vi "Enter_UnRock_Data.vi"() -> ()   [LabVIEW 2019]
uses:
  Calibration.ctl
  <vilib>/Utility/NIReport.llb/Report Type.ctl
  <vilib>/addons/database/Connection.llb/DB Tools Open Connec (Path).vi
  <vilib>/addons/_office/word.llb/Word Find & Replace (str).vi
  <vilib>/addons/database/_DB Variant To Data/Database Variant To Data.xnode
  <vilib>/Utility/NIReport.llb/NI_report.lvclass
  <vilib>/addons/database/NI_Database_API.lvlib
  TEST.lvclass
  <vilib>/Utility/NIReport.llb/NI_ReportGenerationCore.lvlib
  <vilib>/addons/_office/NI_ReportGenerationToolkit.lvlib
  <vilib>/Utility/NIReport.llb/Word/NI_Word.lvclass
panel:
  in  "校准日期":timestamp format="%<%Y/%m/%d>T"
  in  "生产日期":timestamp format="%<%Y/%m/%d>T"
  in  "批号":string
  in  "data":sgl[][](array[numeric]) format="%#.4g"
  out "初始化成功":bool
  out "error out":errorcluster
  in  "init":bool
  in  "NAME":string
  out "HS2":string[](array[string])
  out "CFXWC":string[](array[string])
  out "HAWC":string[](array[string])
  out "允许误差%":string[](array[string])
  out "试验力N(kg/g)":string[](array[string])
  out "执行状态":bool
  out "数据写入成功":bool
  in  "print_calibration":bool
  in  "print_data":bool
  in  "核验员":string
  in  "tsd":sgl[](array[numeric])=[1.0, 1.0, 1.0, 1.0] format="%#.4g"
  in  "停止":bool
  in  "write":bool
  in  "clear":bool
  in  "TEMP":string
  in  "TSN":string
  in  "MODE":string
  out "REP":sgl[](array[numeric]) format="%#.2g"
  out "HV":sgl[](array[numeric]) format="%#.2g"
  out "AVG":sgl[](array[numeric]) format="%#.2g"
  in  "TV":sgl[][](array[numeric]) format="%#.2g"
  in  "HS":sgl[](array[numeric])=[0.0, 0.0, 0.0, 0.0, 0.0] format="%#.2g"
  in  "HN":string[](array[string])
  in  "DIN":string
  out "Inacc":sgl[](array[numeric]) format="%#.2g"
  out "Dev":sgl[](array[numeric]) format="%#.4g"
  # "产品名称(首填)："
  # "型号："
  # "制造编号："
  # "温度："
  # "℃"
  # "试验力测试"
  # "最大偏差"
  # "误差%"
  # "2"
  # "3"
  # "1"
  # "测试力标准值"
  # "±"
  # "±"
  # "±"
  # "±"
  # "±"
  # "±"
  # "±"
  # "±"
  # "硬度测试"
  # "金刚石压头编号："
  # "测试值"
  # "硬度块\n标准值"
  # "硬度块\n  编号"
  # "硬度值"
  # "重复性"
  # "平均值"
  # "1"
  # "2"
  # "4"
  # "5"
  # "3"
  # "实际误差"
  # "允许误差"
  # "实际误差"
  # "允许误差"
  # "±1.0"
  # "1.0RA"
  # "RA"
  # "±1.5"
  # "1.5RB"
  # "RB"
  # "±1.5"
  # "1.5RC"
  # "RC"
  # "±1.2"
  # "1.2RC"
  # "RC"
  # "±1.0"
  # "1.2RC"
  # "RC"
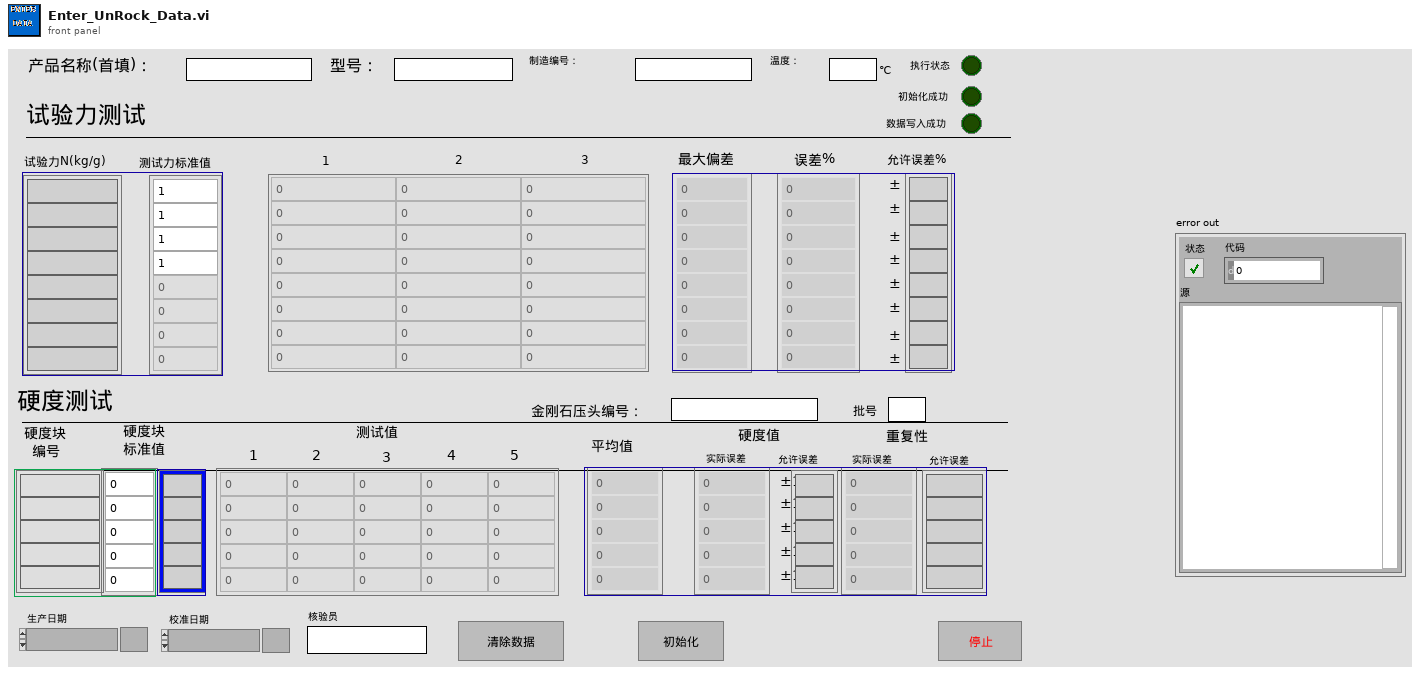
[diagram p1: front panel]
types:
  T1 = enum8{"Enabled", "Disabled", "Disabled and Grayed Out"}
  T2 = enum16{"open", "replace", "create", "open or create", "replace or create", "replace or create with confirmation"}
  T3 = typedef "TEST.lvclass/Calibration.ctl" = cluster{"NAM":string, "MODE":string, "TSN":string, "TDN":string, "DIN":string, "PROD":string, "CALD":string, "REV":string}
  T4 = typedef "NI_ReportGenerationCore.lvlib/Report Type.ctl" = enum16{"HTML", "Word", "Excel"}
  T5 = enum16{"maximized", "minimized", "normal", "no change"}
  T6 = typedef "NI_Database_API.lvlib/Conn ObjectReference.ctl" = refnum<k1>
  T7 = typedef "NI_Database_API.lvlib/DB Tools DataTypes.ctl" = enum16{"String", "Long (I32)", "Single (SGL)", "Double (DBL)", "Date/Time", "Binary"}
  T8 = cluster{"name":string, "database data type":T7, "defined size":i32}[]
  T9 = cluster{"name":string, "database data type":T7, "defined size":i32, bool}
  T10 = typedef "TEST.lvclass/Unrock_Cluster.ctl" = cluster{"MODE":string, "TSN":string, "Temp":string, "Test_load_row1":T11, "Test_load_row2":T11, "Test_load_row3":T11, "Test_load_row4":T11, "Test_load_row5":T11, "Test_load_row6":T11, "Test_load_row7":T11, "Test_load_row8":T11, "DIN":string, "Hardness_test_row1":T12, "Hardness_test_row2":T12, "Hardness_test_row3":T12, "Hardness_test_row4":T12, "Hardness_test_row5":T12}
  T11 = typedef "TEST.lvclass/Test_load.ctl" = cluster{"TEST1":sgl, "TEST2":sgl, "TEST3":sgl, "DEV":sgl, "INACC":sgl}
  T12 = typedef "TEST.lvclass/Hardness_test.ctl" = cluster{"HN":string, "HS":sgl, "TV1":sgl, "TV2":sgl, "TV3":sgl, "TV4":sgl, "TV5":sgl, "AVG":sgl, "HV":sgl, "REP":sgl}
  T13 = typedef "TEST.lvclass/Unrock_Data.ctl" = cluster{"MOD":string, "TSN":string, "Temp":string, "TEST1":sgl, "TEST2":sgl, "TEST3":sgl, "DEV":sgl, "INACC":sgl, "TEST1":sgl, "TEST2":sgl, "TEST3":sgl, "DEV":sgl, "INACC":sgl, "TEST1":sgl, "TEST2":sgl, "TEST3":sgl, "DEV":sgl, "INACC":sgl, "TEST1":sgl, "TEST2":sgl, "TEST3":sgl, "DEV":sgl, "INACC":sgl, "TEST1 5":sgl, "TEST2 5":sgl, "TEST3 5":sgl, "DEV 5":sgl, "INACC 5":sgl, "TEST1 4":sgl, "TEST2 4":sgl, "TEST3 4":sgl, "DEV 4":sgl, "INACC 4":sgl, "TEST1 3":sgl, "TEST2 3":sgl, "TEST3 3":sgl, "DEV 3":sgl, "INACC 3":sgl, "TEST1 2":sgl, "TEST2 2":sgl, "TEST3 2":sgl, "DEV 2":sgl, "INACC 2":sgl, "DIN":string, "HN":string, "HS":sgl, "TV1":sgl, "TV2":sgl, "TV3":sgl, "TV4":sgl, "TV5":sgl, "AVG":sgl, "HV":sgl, "REP":sgl, "HN":string, "HS":sgl, "TV1":sgl, "TV2":sgl, "TV3":sgl, "TV4":sgl, "TV5":sgl, "AVG":sgl, "HV":sgl, "REP":sgl, "HN":string, "HS":sgl, "TV1":sgl, "TV2":sgl, "TV3":sgl, "TV4":sgl, "TV5":sgl, "AVG":sgl, "HV":sgl, "REP":sgl, "HN":string, "HS":sgl, "TV1":sgl, "TV2":sgl, "TV3":sgl, "TV4":sgl, "TV5":sgl, "AVG":sgl, "HV":sgl, "REP":sgl, "HN":string, "HS":sgl, "TV1":sgl, "TV2":sgl, "TV3":sgl, "TV4":sgl, "TV5":sgl, "AVG":sgl, "HV":sgl, "REP":sgl, "NAM":string, "TDN":string, "PROD":string, "CALD":string, "REV":string}
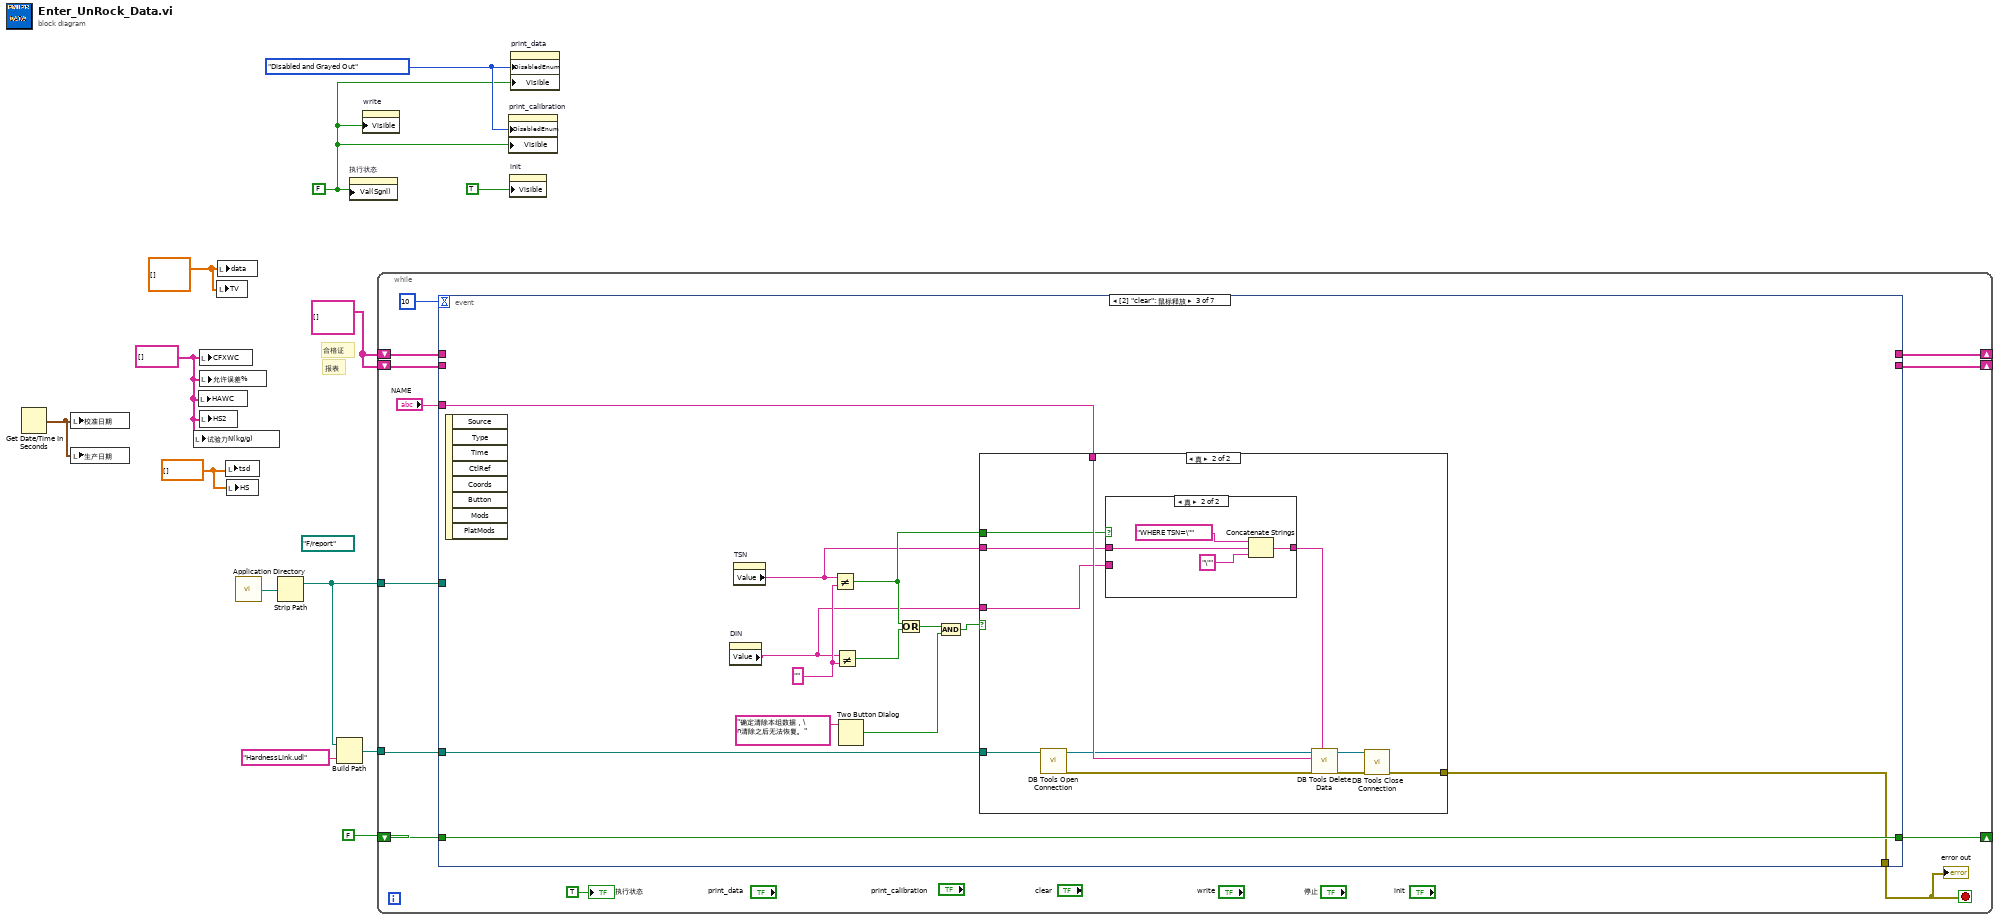
[diagram p0: block diagram]
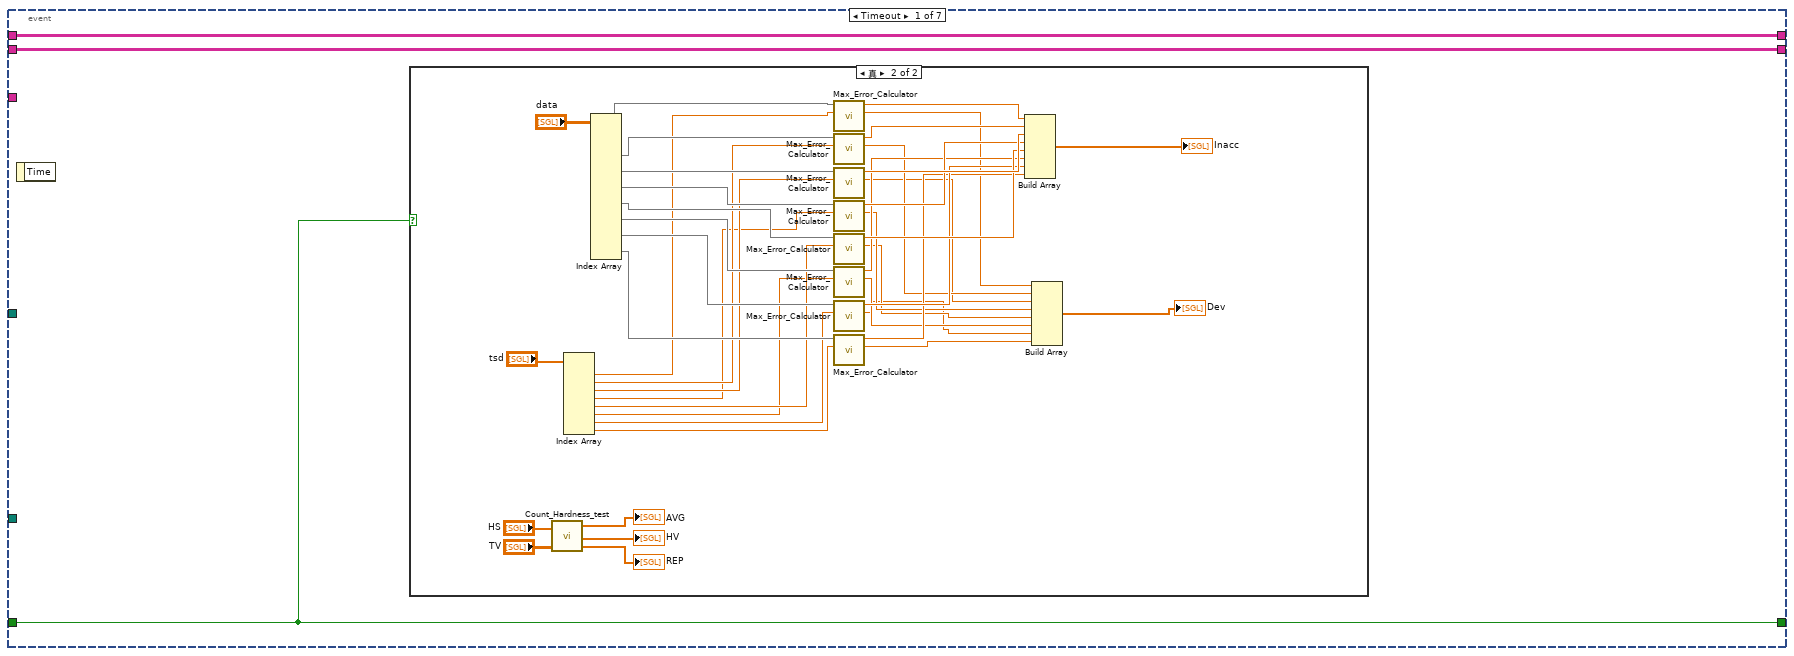
[diagram p2: hidden frame]
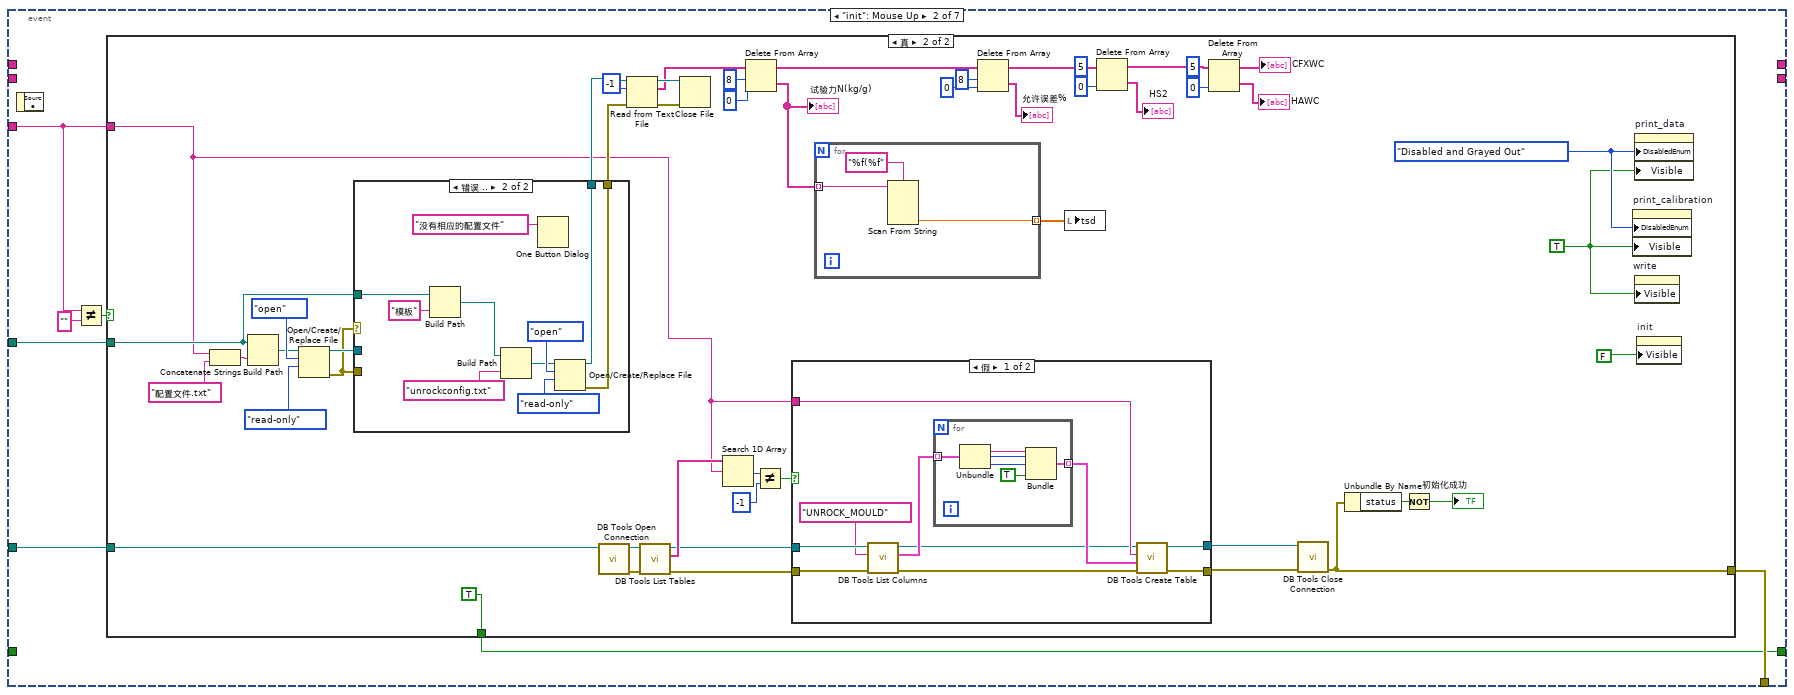
[diagram p4: hidden frame]
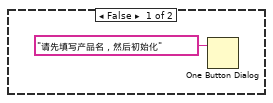
[diagram p5: hidden frame]
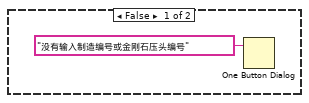
[diagram p8: hidden frame]
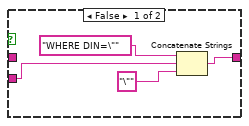
[diagram p9: hidden frame]
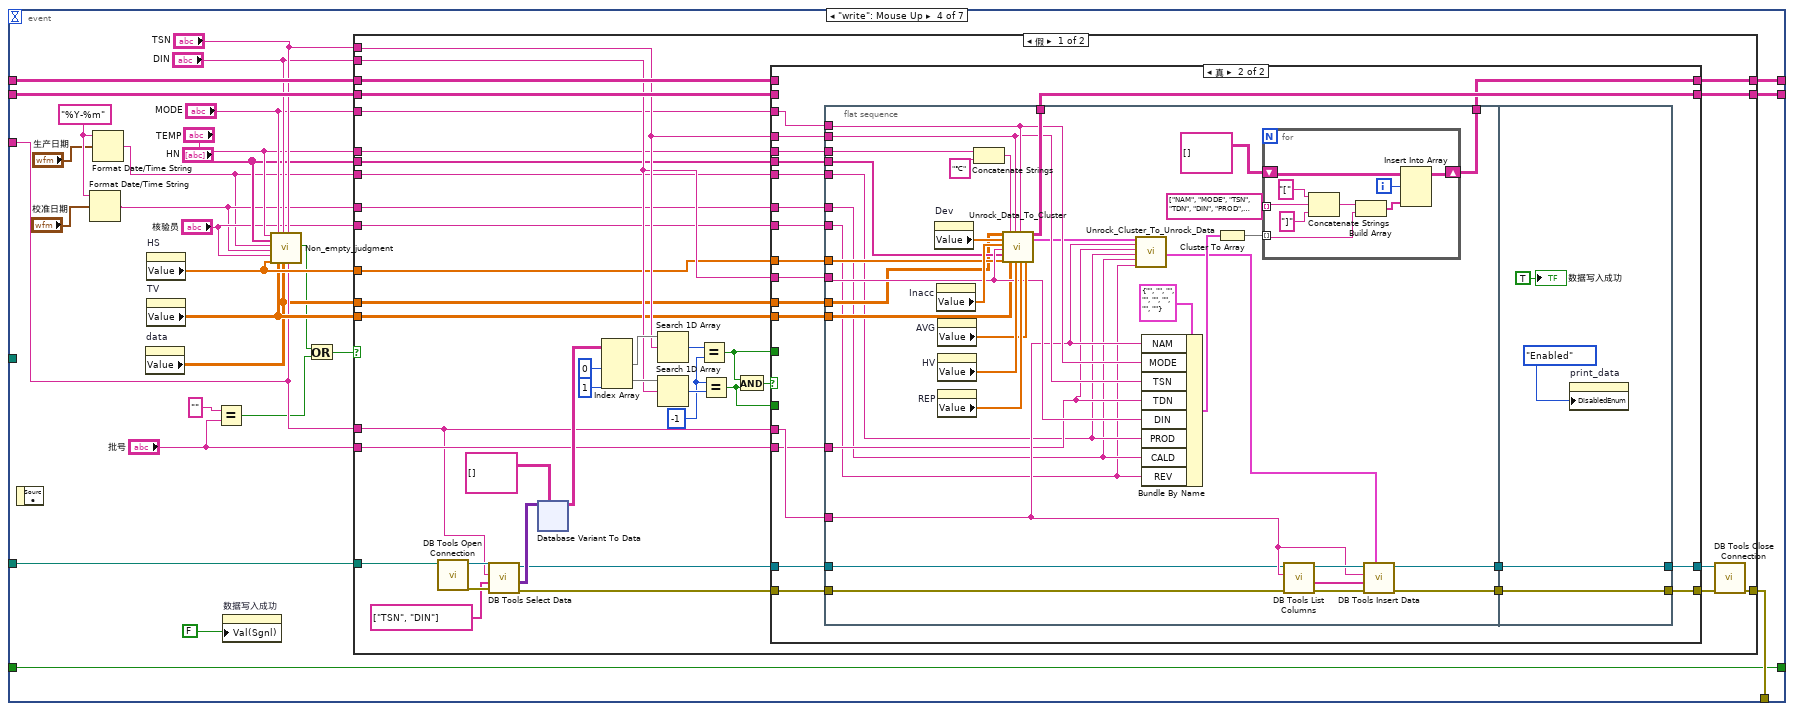
[diagram p10: hidden frame]
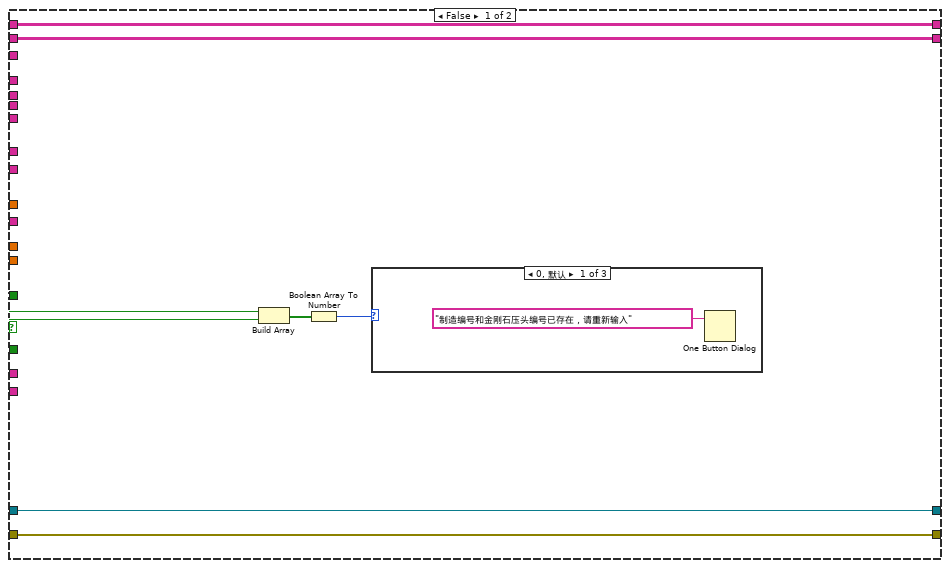
[diagram p11: hidden frame]
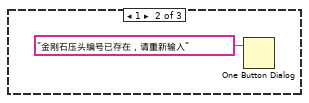
[diagram p12: hidden frame]
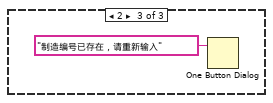
[diagram p13: hidden frame]
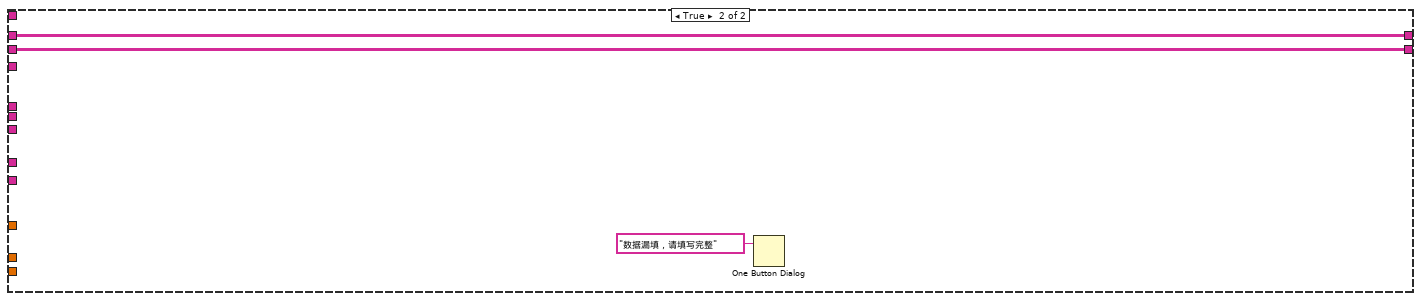
[diagram p14: hidden frame]
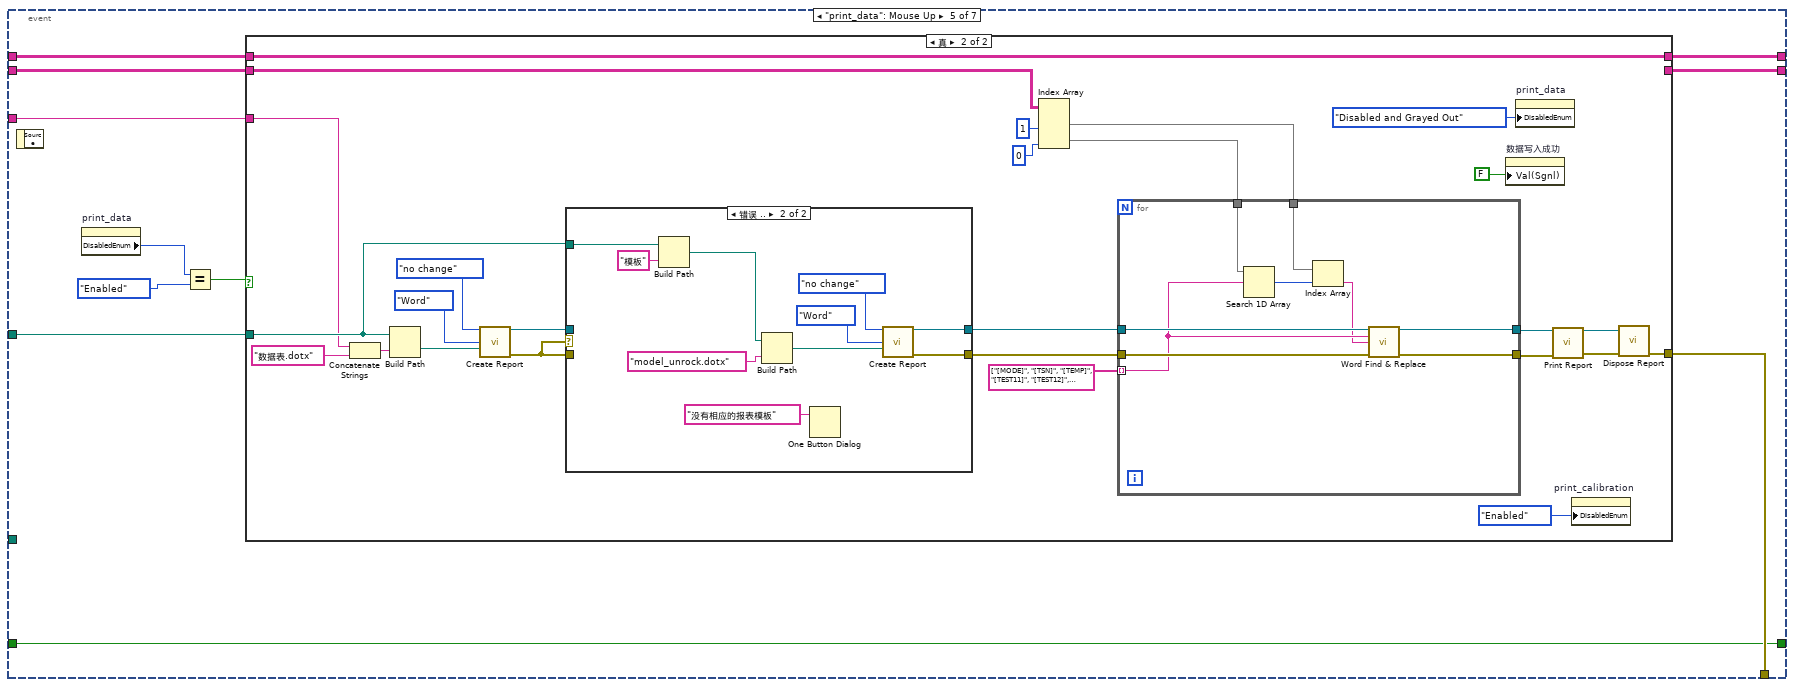
[diagram p15: hidden frame]
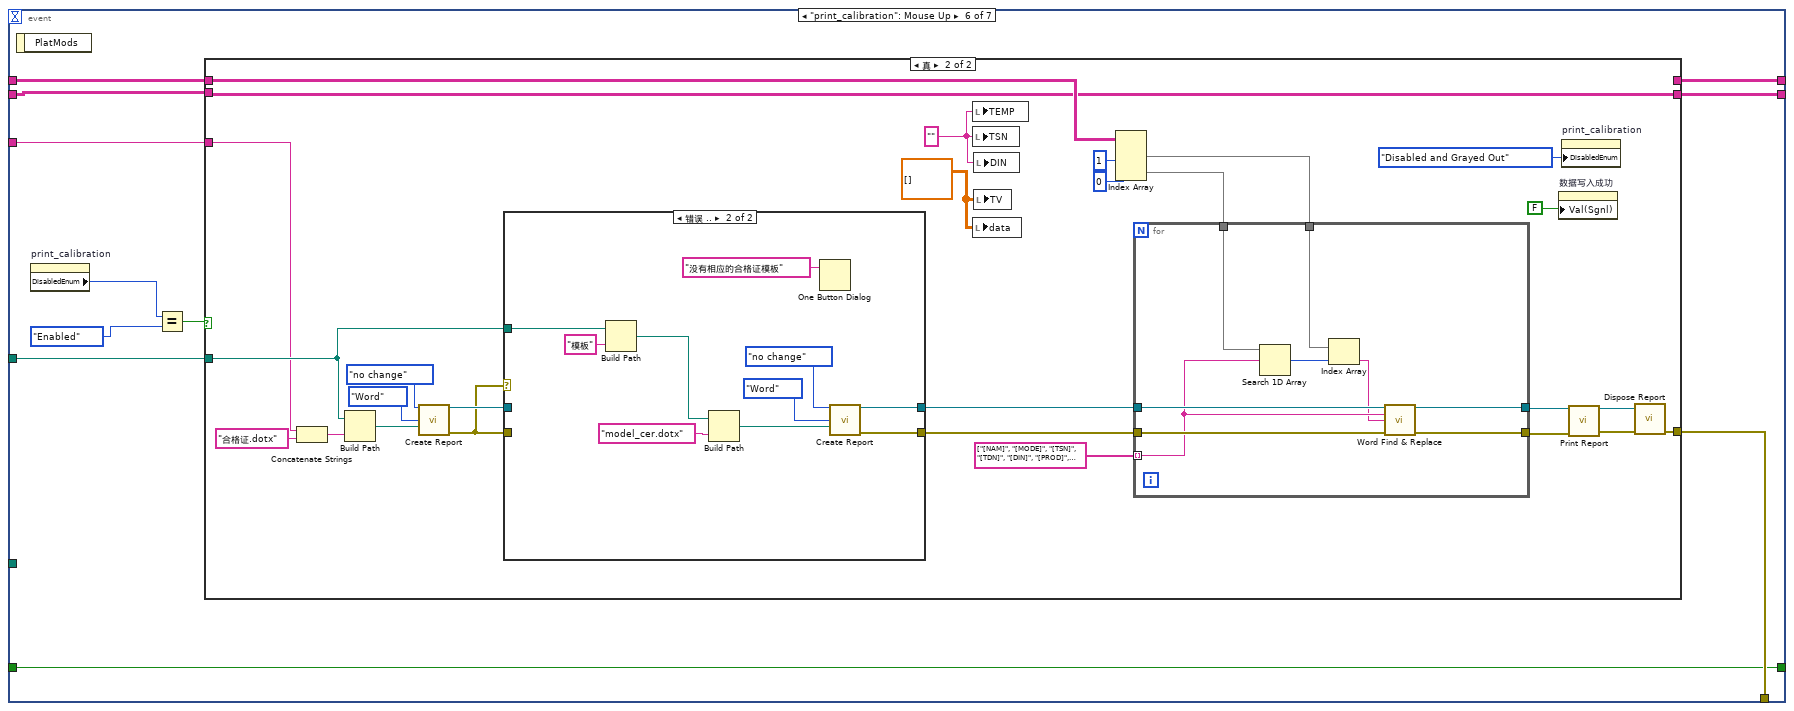
[diagram p18: hidden frame]
diagram:
  w6 = dbl[][] []
  w7 = sgl[] []
  w9 = string[] []
  (unwired) path "F:/report" ("data__in")
  w10 = FALSE
  w13 = T1."Disabled and Grayed Out" ("禁用")
  w12 = string[][] []
  # "报表"
  # "合格证"
  n1 = Get Date/Time In Seconds() -> (seconds since 1Jan1904=w1:timestamp)
  n2 = local write "校准日期"(w1) -> ()
  n3 = local write "生产日期"(w1) -> ()
  n4 = local write "试验力N(kg/g)"(w9) -> ()
  n5 = local write "HAWC"(w9) -> ()
  n6 = local write "CFXWC"(w9) -> ()
  n7 = local write "允许误差%"(w9) -> ()
  n8 = local write "HS2"(w9) -> ()
  n9 = local write "TV"(w6) -> ()
  n10 = local write "data"(w6) -> ()
  n11 = local write "tsd"(w7) -> ()
  n12 = local write "HS"(w7) -> ()
  n13 = call <vilib>:"Application Directory.vi"() -> ("Application Directory"=w5:path)
  n14 = Strip Path(path=w5) -> (stripped path=w2:path)  [unwired: 1 out]
  n15 = Build Path(base path=w2, name or relative path="HardnessLink.udl" ("名称或相对路径")) -> (appended path=w3:path)
  n16 = property on="执行状态" class="Bool (严格)"("Val(Sgnl)"=w10) -> ()  [unwired: 2 in, 2 out]
  n17 = property on="write" class="Bool (严格)"("Visible"=w10) -> ()  [unwired: 2 in, 2 out]
  n18 = while {
    shift-right: [w24] -> _
    shift-left: w12 -> [w23]
    shift-right: [w21] -> _
    shift-left: w12 -> [w20]
    tunnel: w2 -> [w15]
    shift-right: [w17] -> _
    shift-left: FALSE -> [w16]
    tunnel: w3 -> [w14]
    stop <- w18 stop-if-true
    n19 = event shown="[2] \"clear\": 鼠标释放" {
      selector: _ -> [_ _ _ _ _ _ _]
      dyn-events: _ -> [_ _ _ _ _ _ _]
      timeout: 10 -> [_ _ _ _ _ _ _]
      tunnel: [_ w75 w167 w217 w399 w459 errorcluster {"status"=TRUE, "code"=0, "source"=""} ("error out")] -> w18
      tunnel: [w28 _ _ w221 w391 w453 _] -> w24
      tunnel: w23 -> [w28 _ _ w218 w395 w454 _]
      tunnel: [w27 _ _ w220 w389 w452 _] -> w21
      tunnel: w20 -> [w27 _ _ w219 w390 w455 _]
      tunnel: "NAME" -> [_ w74 w169 w208 w397 w456 _]
      tunnel: w15 -> [_ w76 _ _ w398 w458 _]
      tunnel: [w26 w71 w173 w207 w396 w457 FALSE] -> w17
      tunnel: w16 -> [w26 _ w173 w207 w396 w457 _]
      tunnel: w14 -> [_ w70 w168 w199 _ _ _]
      event Timeout {
        n20 = event-data() -> ()  [unwired: 1 in, 1 out]
        n21 = case shown="真" w26 {
          frame False {
          }
          frame True {
            n22 = call "Count_Hardness_test.vi"("HS"="HS", "TV"="TV") -> ("AVG"=→"AVG":sgl[], "HV"=→"HV":sgl[], "REP"=→"REP":sgl[])
            n23 = Index Array(array="tsd") -> (element #1=w54:sgl, element #2=w53:sgl, element #3=w52:sgl, element #4=w51:sgl, element #5=w50:sgl, element #6=w49:sgl, element #7=w48:sgl, element #8=w47:sgl)  [unwired: 8 in]
            n24 = Index Array(array="data") -> (element #1=w63:sgl[], element #2=w62:sgl[], element #3=w61:sgl[], element #4=w60:sgl[], element #5=w59:sgl[], element #6=w58:sgl[], element #7=w57:sgl[], element #8=w56:sgl[])  [unwired: 16 in]
            n25 = call "Max_Error_Calculator.vi"("数值"=w54, "数组"=w63) -> ("dev"=w37:sgl, "inaccc"=w46:sgl)  [unwired: 8 in]
            n26 = call "Max_Error_Calculator.vi"("数值"=w53, "数组"=w62) -> ("dev"=w36:sgl, "inaccc"=w45:sgl)  [unwired: 8 in]
            n27 = call "Max_Error_Calculator.vi"("数值"=w52, "数组"=w61) -> ("dev"=w35:sgl, "inaccc"=w44:sgl)  [unwired: 8 in]
            n28 = call "Max_Error_Calculator.vi"("数值"=w51, "数组"=w60) -> ("dev"=w34:sgl, "inaccc"=w43:sgl)  [unwired: 8 in]
            n29 = call "Max_Error_Calculator.vi"("数值"=w50, "数组"=w59) -> ("dev"=w33:sgl, "inaccc"=w42:sgl)  [unwired: 8 in]
            n30 = call "Max_Error_Calculator.vi"("数值"=w49, "数组"=w58) -> ("dev"=w32:sgl, "inaccc"=w41:sgl)  [unwired: 8 in]
            n31 = call "Max_Error_Calculator.vi"("数值"=w48, "数组"=w57) -> ("dev"=w31:sgl, "inaccc"=w40:sgl)  [unwired: 8 in]
            n32 = call "Max_Error_Calculator.vi"("数值"=w47, "数组"=w56) -> ("dev"=w30:sgl, "inaccc"=w39:sgl)  [unwired: 8 in]
            n33 = Build Array(w46, w45, w44, w43, w42, w41, w40, w39) -> (→"Inacc":sgl[])
            n34 = Build Array(w37, w36, w35, w34, w33, w32, w31, w30) -> (→"Dev":sgl[])
          }
        }
      }
      event "init": Mouse Up {
        n35 = event-data() -> ()  [unwired: 1 in, 1 out]
        n36 = Not Equal?(x=w74, y="" ("NAME")) -> (x != y?=w72:bool)
        n37 = case shown="真" w72 {
          tunnel: w70 -> [_ w127]
          tunnel: w76 -> [_ w90]
          tunnel: [_ w89] -> w75
          tunnel: w74 -> [_ w78]
          tunnel: [_ TRUE] -> w71
          frame False {
            n38 = One Button Dialog(message="请先填写产品名，然后初始化" ("消息")) -> ()  [unwired: 1 in, 1 out]
          }
          frame True {
            w115 = T1."Disabled and Grayed Out" ("禁用")
            w114 = TRUE ("可见")
            n39 = Concatenate Strings(w78, "配置文件.txt" ("名称或相对路径")) -> (w95:string)
            n40 = Build Path(base path=w90, name or relative path=w95) -> (appended path=w108:path)
            n41 = Open/Create/Replace File(file path (use dialog)=w108, operation (0:open)=T2."open" ("操作(0:open)"), access (0:read/write)=enum16{"read/write", "read-only", "write-only"}."read-only" ("权限(0:read/write)")) -> (refnum out=w93:refnum<file>, error out=w91:errorcluster)  [unwired: 3 in, 1 out]
            n42 = case shown="错误 .." w91 {
              tunnel: [w132 w142] -> w94
              tunnel: w93 -> [w132 _]
              tunnel: [w131 w141] -> w92
              tunnel: w91 -> [w131 _]
              tunnel: w90 -> [_ w136]
              frame No Error {
              }
              frame Error {
                n43 = Build Path(base path=w136, name or relative path="模板" ("名称或相对路径")) -> (appended path=w134:path)
                n44 = Build Path(base path=w134, name or relative path="unrockconfig.txt") -> (appended path=w138:path)
                n45 = One Button Dialog(message="没有相应的配置文件" ("消息")) -> ()  [unwired: 1 in, 1 out]
                n46 = Open/Create/Replace File(file path (use dialog)=w138, operation (0:open)=T2."open" ("操作(0:open)"), access (0:read/write)=enum16{"read/write", "read-only", "write-only"}."read-only" ("权限(0:read/write)")) -> (refnum out=w142:refnum<file>, error out=w141:errorcluster)  [unwired: 3 in, 1 out]
              }
            }
            n47 = call-poly <vilib>:"DB Tools Open Connection.vi"("connection information"=w127) -> ("error out"=w125:errorcluster, "connection reference"=w126:T6)  [unwired: 7 in]
            n48 = Read from Text File(file (use dialog)=w94, count=-1 ("计数"), error in=w92) -> (refnum out=w110:refnum<file>, text=w107:string[], error out=w111:errorcluster)  [unwired: 1 in, 1 out]
            n49 = call <vilib>:"DB Tools List Tables.vi"("error in (no error)"=w125, "connection reference"=w126) -> ("error out"=w119:errorcluster, "tables"=w124:string[], "connection reference out"=w120:T6)  [unwired: 3 in]
            n50 = Close File(refnum=w110, error in=w111) -> ()  [unwired: 2 out]
            n51 = Search 1D Array(1D array=w124, element=w78) -> (index of element=w123:i32)  [unwired: 1 in]
            n52 = Delete From Array(array=w107, length=8 ("长度"), index=0 ("索引")) -> (deleted portion=w85:string[], array with subset deleted=w79:string[])
            "试验力N(kg/g)" <- w85
            n53 = Not Equal?(x=w123, y=-1) -> (x != y?=w121:bool)
            n54 = case shown="假" w121 {
              tunnel: [w144 w160] -> w117
              tunnel: w120 -> [w152 w160]
              tunnel: w119 -> [w151 w159]
              tunnel: [w143 w159] -> w118
              tunnel: w78 -> [w147 _]
              frame False {
                n55 = call <vilib>:"DB Tools List Columns.vi"("error in (no error)"=w151, "table"="UNROCK_MOULD", "connection reference"=w152) -> ("error out"=w145:errorcluster, "column information"=w149:T8, "connection reference out"=w146:T6)  [unwired: 1 in, 1 out]
                n56 = for {
                  tunnel: w149 -> [w158] mode=indexing
                  tunnel: [w153] -> w148 mode=indexing
                  n57 = Unbundle(w158) -> ("name"=w157:string, "database data type"=w156:T7, "defined size"=w155:i32)
                  n58 = Bundle("name"=w157, "database data type"=w156, "defined size"=w155, TRUE) -> (w153:T9)  [unwired: 1 in]
                }
                n59 = call <vilib>:"DB Tools Create Table.vi"("error in (no error)"=w145, "column information"=w148, "table"=w147, "connection reference"=w146) -> ("error out"=w143:errorcluster, "connection reference out"=w144:T6)  [unwired: 4 in]
              }
              frame True {
              }
            }
            n60 = for {
              tunnel: w85 -> [w129] mode=indexing
              tunnel: [w128] -> w86 mode=indexing
              n61 = Scan From String(format string="%f(%f" ("格式字符串"), input string=w129) -> (output 2=w128:dbl)  [unwired: 5 in, 3 out]
            }
            n62 = Delete From Array(array=w79, length=8 ("长度"), index=0 ("索引")) -> (deleted portion=→"允许误差%":string[], array with subset deleted=w102:string[])
            n63 = local write "tsd"(w86) -> ()
            n64 = Delete From Array(array=w102, length=5 ("长度"), index=0 ("索引")) -> (deleted portion=→"HS2":string[], array with subset deleted=w99:string[])
            n65 = Delete From Array(array=w99, length=5 ("长度"), index=0 ("索引")) -> (deleted portion=→"HAWC":string[], array with subset deleted=→"CFXWC":string[])
            n66 = call <vilib>:"DB Tools Close Connection.vi"("error in (no error)"=w118, "connection reference"=w117) -> ("error out"=w89:errorcluster)  [unwired: 5 in]
            n67 = Unbundle By Name(w89) -> ("status"=w88:bool)
            n68 = Not(x=w88) -> (.not. x?=→"初始化成功":bool)
            n69 = property on="print_calibration" class="Bool (严格)"("DisabledEnum"=w115, "Visible"=w114) -> ()  [unwired: 2 in, 2 out]
            n70 = property on="print_data" class="Bool (严格)"("DisabledEnum"=w115, "Visible"=w114) -> ()  [unwired: 2 in, 2 out]
            n71 = property on="write" class="Bool (严格)"("Visible"=w114) -> ()  [unwired: 2 in, 2 out]
            n72 = property on="init" class="Bool (严格)"("Visible"=FALSE ("可见")) -> ()  [unwired: 2 in, 2 out]
          }
        }
      }
      event "clear": Mouse Up {
        w172 = ""
        n73 = event-data() -> ()  [unwired: 1 in, 8 out]
        n74 = property on="DIN" class="Str"() -> ("Value"=w165:string)  [unwired: 2 in, 2 out]
        n75 = property on="TSN" class="Str"() -> ("Value"=w166:string)  [unwired: 2 in, 2 out]
        n76 = Not Equal?(x=w166, y=w172) -> (x != y?=w170:bool)
        n77 = Not Equal?(x=w165, y=w172) -> (x != y?=w171:bool)
        n78 = Two Button Dialog(message="确定清除本组数据，\n清除之后无法恢复。" ("消息")) -> (T button?=w161:bool)  [unwired: 2 in]
        n79 = Or(x=w170, y=w171) -> (x .or. y?=w163:bool)
        n80 = And(x=w163, y=w161) -> (x .and. y?=w162:bool)
        n81 = case shown="真" w162 {
          tunnel: w168 -> [_ w185]
          tunnel: w169 -> [_ w184]
          tunnel: [_ w183] -> w167
          tunnel: w166 -> [_ w177]
          tunnel: w170 -> [_ w176]
          tunnel: w165 -> [_ w175]
          frame False {
            n82 = One Button Dialog(message="没有输入制造编号或金刚石压头编号" ("消息")) -> ()  [unwired: 1 in, 1 out]
          }
          frame True {
            n83 = call-poly <vilib>:"DB Tools Open Connection.vi"("connection information"=w185) -> ("error out"=w181:errorcluster, "connection reference"=w182:T6)  [unwired: 7 in]
            n84 = case shown="真" w176 {
              tunnel: [w187 w191] -> w178
              tunnel: w177 -> [_ w190]
              tunnel: w175 -> [w186 _]
              frame False {
                n85 = Concatenate Strings("WHERE DIN=\"", w186, "\"" ("字符串")) -> (w187:string)
              }
              frame True {
                n86 = Concatenate Strings("WHERE TSN=\"", w190, "\"" ("字符串")) -> (w191:string)
              }
            }
            n87 = call <vilib>:"DB Tools Delete Data.vi"("condition"=w178, "error in (no error)"=w181, "table"=w184, "connection reference"=w182) -> ("error out"=w180:errorcluster, "connection reference out"=w179:T6)  [unwired: 6 in]
            n88 = call <vilib>:"DB Tools Close Connection.vi"("error in (no error)"=w180, "connection reference"=w179) -> ("error out"=w183:errorcluster)  [unwired: 5 in]
          }
        }
      }
      event "write": Mouse Up {
        w198 = "%Y-%m" ("时间格式字符串(%c)")
        n89 = event-data() -> ()  [unwired: 1 in, 1 out]
        n90 = Format Date/Time String(time format string (%c)=w198, seconds (now)="校准日期") -> (date/time string=w195:string)  [unwired: 1 in]
        n91 = Format Date/Time String(time format string (%c)=w198, seconds (now)="生产日期") -> (date/time string=w194:string)  [unwired: 1 in]
        n92 = property on="data" class="Arr (严格)"() -> ("Value"=w205:sgl[][])  [unwired: 2 in, 2 out]
        n93 = property on="HS" class="Arr (严格)"() -> ("Value"=w210:sgl[])  [unwired: 2 in, 2 out]
        n94 = property on="TV" class="Arr (严格)"() -> ("Value"=w209:sgl[][])  [unwired: 2 in, 2 out]
        n95 = Equal?(x="", y="批号") -> (x = y?=w200:bool)
        n96 = property on="数据写入成功" class="Bool (严格)"("Val(Sgnl)"=FALSE) -> ()  [unwired: 2 in, 2 out]
        n97 = call "Non_empty_judgment.vi"("TEMP"="TEMP", "HN"="HN", "生产日期"=w194, "校准日期"=w195, "核验员"="核验员", "HS"=w210, "MODE"="MODE", "TV"=w209, "DIN"="DIN", "TESTS"=w205, "TSN"="TSN", "NAME"=w208) -> ("结果"=w201:bool)  [unwired: 7 in]
        n98 = Or(x=w201, y=w200) -> (x .or. y?=w202:bool)
        n99 = case shown="假" w202 {
          tunnel: [w260 w387] -> w221
          tunnel: [w259 w388] -> w220
          tunnel: w219 -> [w244 w388]
          tunnel: w218 -> [w243 w387]
          tunnel: w199 -> [w242 _]
          tunnel: [w235 _] -> w217
          tunnel: "TSN" -> [w234 _]
          tunnel: "DIN" -> [w233 _]
          tunnel: "MODE" -> [w232 _]
          tunnel: "TEMP" -> [w231 _]
          tunnel: "HN" -> [w230 _]
          tunnel: w194 -> [w229 _]
          tunnel: w195 -> [w228 _]
          tunnel: "核验员" -> [w227 _]
          tunnel: w210 -> [w226 _]
          tunnel: w209 -> [w225 _]
          tunnel: w208 -> [w222 _]
          tunnel: w205 -> [w224 _]
          tunnel: "批号" -> [w223 _]
          frame False {
            w246 = -1
            n100 = call-poly <vilib>:"DB Tools Open Connection.vi"("connection information"=w242) -> ("error out"=w257:errorcluster, "connection reference"=w258:T6)  [unwired: 7 in]
            n101 = call <vilib>:"DB Tools Select Data.vi"("error in (no error)"=w257, "columns"=string[] ["TSN", "DIN"], "table"=w222, "connection reference"=w258) -> ("error out"=w238:errorcluster, "data"=w255:variant[][], "connection reference out"=w239:T6)  [unwired: 2 in]
            n102 = xnode "Database Variant To Data"("database variant"=w255, "type"=string[][] []) -> ("data"=w253:string[][])  [unwired: 1 in, 1 out]
            n103 = Index Array(array=w253, index (col) #1=0 ("禁用的索引 (列)"), index (col) #2=1 ("索引 (列)")) -> (element #1=w250:string[], element #2=w249:string[])  [unwired: 2 in]
            n104 = Search 1D Array(1D array=w250, element=w234) -> (index of element=w248:i32)  [unwired: 1 in]
            n105 = Search 1D Array(1D array=w249, element=w233) -> (index of element=w247:i32)  [unwired: 1 in]
            n106 = Equal?(x=w248, y=w246) -> (x = y?=w241:bool)
            n107 = Equal?(x=w246, y=w247) -> (x = y?=w240:bool)
            n108 = And(x=w241, y=w240) -> (x .and. y?=w245:bool)
            n109 = case shown="真" w245 {
              tunnel: [w267 w292] -> w260
              tunnel: [w268 w291] -> w259
              tunnel: w234 -> [_ w290]
              tunnel: w233 -> [_ w289]
              tunnel: w244 -> [w268 _]
              tunnel: w243 -> [w267 _]
              tunnel: w222 -> [_ w288]
              tunnel: w241 -> [w265 _]
              tunnel: w240 -> [w266 _]
              tunnel: w239 -> [w262 w287]
              tunnel: w238 -> [w261 w286]
              tunnel: [w262 w284] -> w237
              tunnel: [w261 w282] -> w236
              tunnel: w232 -> [_ w281]
              tunnel: w231 -> [_ w280]
              tunnel: w230 -> [_ w279]
              tunnel: w229 -> [_ w278]
              tunnel: w226 -> [_ w277]
              tunnel: w225 -> [_ w276]
              tunnel: w228 -> [_ w275]
              tunnel: w227 -> [_ w274]
              tunnel: w224 -> [_ w273]
              tunnel: w223 -> [_ w272]
              frame False {
                n110 = Build Array(w265, w266) -> (w264:bool[])
                n111 = Boolean Array To Number(Boolean array=w264) -> (number=w263:u32)
                n112 = case shown="0, 默认" w263 {
                  frame 0, Default {
                    n113 = One Button Dialog(message="制造编号和金刚石压头编号已存在，请重新输入" ("消息")) -> ()  [unwired: 1 in, 1 out]
                  }
                  frame 1 {
                    n114 = One Button Dialog(message="金刚石压头编号已存在，请重新输入" ("消息")) -> ()  [unwired: 1 in, 1 out]
                  }
                  frame 2 {
                    n115 = One Button Dialog(message="制造编号已存在，请重新输入" ("消息")) -> ()  [unwired: 1 in, 1 out]
                  }
                }
              }
              frame True {
                n116 = flat-sequence {
                  tunnel: [w317] -> w292
                  tunnel: [w314] -> w291
                  tunnel: w290 -> [w304]
                  tunnel: w289 -> [w312]
                  tunnel: w288 -> [w299]
                  tunnel: w287 -> [w294]
                  tunnel: w286 -> [w293]
                  tunnel: [w311] -> w285
                  tunnel: [w310] -> w283
                  tunnel: w281 -> [w305]
                  tunnel: w280 -> [w309]
                  tunnel: w279 -> [w308]
                  tunnel: w278 -> [w297]
                  tunnel: w277 -> [w307]
                  tunnel: w276 -> [w306]
                  tunnel: w275 -> [w296]
                  tunnel: w274 -> [w295]
                  tunnel: w273 -> [w303]
                  tunnel: w272 -> [w298]
                  tunnel: w285 -> [w340]
                  tunnel: [w340] -> w284
                  tunnel: w283 -> [w339]
                  tunnel: [w339] -> w282
                  frame #0 {
                    n117 = property on="Dev" class="Arr (严格)"() -> ("Value"=w325:sgl[])  [unwired: 2 in, 2 out]
                    n118 = property on="Inacc" class="Arr (严格)"() -> ("Value"=w324:sgl[])  [unwired: 2 in, 2 out]
                    n119 = property on="AVG" class="Arr (严格)"() -> ("Value"=w321:sgl[])  [unwired: 2 in, 2 out]
                    n120 = property on="HV" class="Arr (严格)"() -> ("Value"=w323:sgl[])  [unwired: 2 in, 2 out]
                    n121 = property on="REP" class="Arr (严格)"() -> ("Value"=w322:sgl[])  [unwired: 2 in, 2 out]
                    n122 = Concatenate Strings(w309, "℃") -> (w319:string)
                    n123 = call "Unrock_Data_To_Cluster.vi"("Test"=w303, "Dev"=w325, "Inacc"=w324, "DIN"=w312, "HN"=w308, "HS"=w307, "TEMP"=w319, "TV"=w306, "TSN"=w304, "HV"=w323, "MODE"=w305, "REP"=w322, "AVG"=w321) -> ("All_data_String"=w317:string[][], "输出簇"=w301:T10)  [unwired: 5 in]
                    n124 = call "Unrock_Cluster_To_Unrock_Data.vi"("Unrock_Cluster"=w301, "NAM"=w299, "TDN"=w298, "PROD"=w297, "CALD"=w296, "REV"=w295) -> ("Cluster67"=w302:T13)  [unwired: 13 in]
                    n125 = Bundle By Name(cluster=T3 {"NAM"="", "MODE"="", "TSN"="", "TDN"="", "DIN"="", "PROD"="", "CALD"="", "REV"=""} ("Cal"), "NAM"=w299, "MODE"=w305, "TSN"=w304, "TDN"=w298, "DIN"=w312, "PROD"=w297, "CALD"=w296, "REV"=w295) -> (w313:T3)
                    n126 = Cluster To Array(cluster=w313) -> (array=w316:string[])
                    n127 = for {
                      tunnel: w316 -> [w337] mode=indexing
                      tunnel: string[] ["NAM", "MODE", "TSN", "TDN", "DIN", "PROD", "CALD", "REV"] ("columns 3") -> [w331] mode=indexing
                      shift-right: [w335] -> w314
                      shift-left: string[][] [] -> [w336]
                      i -> [w334]
                      n128 = Concatenate Strings("[" ("字符串"), w331, "]" ("字符串")) -> (w330:string)
                      n129 = Build Array(w330, w337) -> (w329:string[])
                      n130 = Insert Into Array(array=w336, index (row)=w334, new element=w329) -> (w335:string[][])  [unwired: 1 in]
                    }
                    n131 = call <vilib>:"DB Tools List Columns.vi"("error in (no error)"=w293, "table"=w299, "connection reference"=w294) -> ("error out"=w328:errorcluster, "columns"=w327:string[], "connection reference out"=w326:T6)  [unwired: 1 in, 1 out]
                    n132 = call <vilib>:"DB Tools Insert Data.vi"("data"=w302, "error in (no error)"=w328, "columns"=w327, "table"=w299, "connection reference"=w326) -> ("error out"=w310:errorcluster, "connection reference out"=w311:T6)  [unwired: 5 in]
                  }
                  frame #1 {
                    n133 = property on="print_data" class="Bool (严格)"("DisabledEnum"=T1."Enabled" ("禁用")) -> ()  [unwired: 2 in, 2 out]
                    "数据写入成功" <- TRUE
                  }
                }
              }
            }
            n134 = call <vilib>:"DB Tools Close Connection.vi"("error in (no error)"=w236, "connection reference"=w237) -> ("error out"=w235:errorcluster)  [unwired: 5 in]
          }
          frame True {
            n135 = One Button Dialog(message="数据漏填，请填写完整" ("消息")) -> ()  [unwired: 1 in, 1 out]
          }
        }
      }
      event "print_data": Mouse Up {
        n136 = event-data() -> ()  [unwired: 1 in, 1 out]
        n137 = property on="print_data" class="Bool (严格)"() -> ("DisabledEnum"=w393:T1)  [unwired: 2 in, 2 out]
        n138 = Equal?(x=w393, y=T1."Enabled" ("禁用")) -> (x = y?=w394:bool)
        n139 = case shown="真" w394 {
          tunnel: [_ w417] -> w399
          tunnel: w398 -> [_ w412]
          tunnel: w397 -> [_ w411]
          tunnel: w395 -> [w401 w408]
          tunnel: [w401 _] -> w391
          tunnel: w390 -> [w400 w403]
          tunnel: [w400 w403] -> w389
          frame False {
          }
          frame True {
            n140 = Concatenate Strings(w411, "数据表.dotx" ("字符串")) -> (w418:string)
            n141 = Build Path(base path=w412, name or relative path=w418) -> (appended path=w420:path)
            n142 = call <vilib>:"Create Report.vi"("window state (normal)"=T5."no change", "report type"=Report_Type."Word", "template (empty)"=w420) -> ("report out"=w413:refnum<class "NI_report.lvclass">, "error out"=w416:errorcluster)  [unwired: 11 in]
            n143 = case shown="错误 .." w416 {
              tunnel: w416 -> [w429 _]
              tunnel: [w429 w437] -> w415
              tunnel: [w428 w436] -> w414
              tunnel: w413 -> [w428 _]
              tunnel: w412 -> [_ w433]
              frame No Error {
              }
              frame Error {
                n144 = Build Path(base path=w433, name or relative path="模板" ("名称或相对路径")) -> (appended path=w431:path)
                n145 = Build Path(base path=w431, name or relative path="model_unrock.dotx") -> (appended path=w434:path)
                n146 = One Button Dialog(message="没有相应的报表模板" ("消息")) -> ()  [unwired: 1 in, 1 out]
                n147 = call <vilib>:"Create Report.vi"("window state (normal)"=T5."no change", "report type"=Report_Type."Word", "template (empty)"=w434) -> ("report out"=w436:refnum<class "NI_report.lvclass">, "error out"=w437:errorcluster)  [unwired: 11 in]
              }
            }
            n148 = Index Array(array=w408, index (col) #1=1 ("禁用的索引 (列)"), index (col) #2=0 ("索引 (列)")) -> (element #1=w404:string[], element #2=w405:string[])  [unwired: 2 in]
            n149 = for {
              tunnel: string[] ["[MODE]", "[TSN]", "[TEMP]", "[TEST11]", "[TEST12]", "[TEST13]", "[DEV1]", "[INACC1]", "[TEST21]", "[TEST22]", "[TEST23]", "[DEV2]", "[INACC2]", "[TEST31]", "[TEST32]", "[TEST33]", "[DEV3]", "[INACC3]", "[TEST41]", "[TEST42]", "[TEST43]", "[DEV4]", "[INACC4]", "[TEST51]", "[TEST52]", "[TEST53]", "[DEV5]", "[INACC5]", "[TEST61]", "[TEST62]", "[TEST63]", "[DEV6]", "[INACC6]", "[TEST71]", "[TEST72]", "[TEST73]", "[DEV7]", "[INACC7]", "[TEST81]", "[TEST82]", "[TEST83]", "[DEV8]", "[INACC8]", "[DIN]", "[HN1]", "[HS1]", "[TV11]", "[TV12]", "[TV13]", "[TV14]", "[TV15]", "[AVG1]", "[HV1]", "[REP1]", "[HN2]", "[HS2]", "[TV21]", "[TV22]", "[TV23]", "[TV24]", "[TV25]", "[AVG2]", "[HV2]", "[REP2]", "[HN3]", "[HS3]", "[TV31]", "[TV32]", "[TV33]", "[TV34]", "[TV35]", "[AVG3]", "[HV3]", "[REP3]", "[HN4]", "[HS4]", "[TV41]", "[TV42]", "[TV43]", "[TV44]", "[TV45]", "[AVG4]", "[HV4]", "[REP4]", "[HN5]", "[HS5]", "[TV51]", "[TV52]", "[TV53]", "[TV54]", "[TV55]", "[AVG5]", "[HV5]", "[REP5]"] ("待写入项") -> [w444] mode=indexing
              tunnel: w414 -> [w448]
              tunnel: [w446] -> w424
              tunnel: w415 -> [w447]
              tunnel: [w445] -> w425
              tunnel: w405 -> [w441]
              tunnel: w404 -> [w440]
              n150 = Search 1D Array(1D array=w441, element=w444) -> (index of element=w443:i32)  [unwired: 1 in]
              n151 = Index Array(array=w440, index=w443) -> (element=w442:string)
              n152 = call-poly <vilib>:"Word Find & Replace.vi"("report in"=w448, "find what?"=w444, "replace with"=w442, "error in (no error)"=w447) -> ("report out"=w446:refnum<class "NI_report.lvclass">, "error out"=w445:errorcluster)  [unwired: 9 in, 1 out]
            }
            n153 = property on="数据写入成功" class="Bool (严格)"("Val(Sgnl)"=FALSE) -> ()  [unwired: 2 in, 2 out]
            n154 = property on="print_data" class="Bool (严格)"("DisabledEnum"=T1."Disabled and Grayed Out" ("禁用")) -> ()  [unwired: 2 in, 2 out]
            n155 = call-dynamic "Print Report.vi"("report in"=w424, "error in (no error)"=w425) -> ("report out"=w422:refnum<class "NI_report.lvclass">, "error out"=w423:errorcluster)  [unwired: 12 in]
            n156 = property on="print_calibration" class="Bool (严格)"("DisabledEnum"=T1."Enabled" ("禁用")) -> ()  [unwired: 2 in, 2 out]
            n157 = call-dynamic "Dispose Report.vi"("report in"=w422, "error in (no error)"=w423) -> ("error out"=w417:errorcluster)  [unwired: 13 in]
          }
        }
      }
      event "print_calibration": Mouse Up {
        n158 = event-data() -> ()  [unwired: 1 in, 1 out]
        n159 = property on="print_calibration" class="Bool (严格)"() -> ("DisabledEnum"=w450:T1)  [unwired: 2 in, 2 out]
        n160 = Equal?(x=w450, y=T1."Enabled" ("禁用")) -> (x = y?=w451:bool)
        n161 = case shown="真" w451 {
          tunnel: [_ w482] -> w459
          tunnel: w458 -> [_ w472]
          tunnel: w456 -> [_ w470]
          tunnel: w455 -> [w461 w467]
          tunnel: w454 -> [w460 w462]
          tunnel: [w460 w462] -> w453
          tunnel: [w461 _] -> w452
          frame False {
          }
          frame True {
            w469 = sgl[][] []
            w468 = ""
            n162 = Concatenate Strings(w470, "合格证.dotx" ("字符串")) -> (w478:string)
            n163 = Build Path(base path=w472, name or relative path=w478) -> (appended path=w479:path)
            n164 = call <vilib>:"Create Report.vi"("window state (normal)"=T5."no change", "report type"=Report_Type."Word", "template (empty)"=w479) -> ("report out"=w475:refnum<class "NI_report.lvclass">, "error out"=w474:errorcluster)  [unwired: 11 in]
            n165 = case shown="错误 .." w474 {
              tunnel: [w490 w493] -> w476
              tunnel: w475 -> [w490 _]
              tunnel: w474 -> [w489 _]
              tunnel: [w489 w492] -> w473
              tunnel: w472 -> [_ w494]
              frame No Error {
              }
              frame Error {
                n166 = Build Path(base path=w494, name or relative path="模板" ("名称或相对路径")) -> (appended path=w495:path)
                n167 = Build Path(base path=w495, name or relative path="model_cer.dotx") -> (appended path=w497:path)
                n168 = One Button Dialog(message="没有相应的合格证模板" ("消息")) -> ()  [unwired: 1 in, 1 out]
                n169 = call <vilib>:"Create Report.vi"("window state (normal)"=T5."no change", "report type"=Report_Type."Word", "template (empty)"=w497) -> ("report out"=w493:refnum<class "NI_report.lvclass">, "error out"=w492:errorcluster)  [unwired: 11 in]
              }
            }
            n170 = local write "TEMP"(w468) -> ()
            n171 = local write "TSN"(w468) -> ()
            n172 = local write "data"(w469) -> ()
            n173 = local write "DIN"(w468) -> ()
            n174 = local write "TV"(w469) -> ()
            n175 = Index Array(array=w467, index (col) #1=1 ("禁用的索引 (列)"), index (col) #2=0 ("索引 (列)")) -> (element #1=w463:string[], element #2=w464:string[])  [unwired: 2 in]
            n176 = for {
              tunnel: string[] ["[NAM]", "[MODE]", "[TSN]", "[TDN]", "[DIN]", "[PROD]", "[CALD]", "[REV]"] ("待写入项 2") -> [w505] mode=indexing
              tunnel: w464 -> [w502]
              tunnel: w476 -> [w509]
              tunnel: [w507] -> w487
              tunnel: w473 -> [w508]
              tunnel: [w506] -> w488
              tunnel: w463 -> [w501]
              n177 = Search 1D Array(1D array=w502, element=w505) -> (index of element=w504:i32)  [unwired: 1 in]
              n178 = Index Array(array=w501, index=w504) -> (element=w503:string)
              n179 = call-poly <vilib>:"Word Find & Replace.vi"("report in"=w509, "find what?"=w505, "replace with"=w503, "error in (no error)"=w508) -> ("report out"=w507:refnum<class "NI_report.lvclass">, "error out"=w506:errorcluster)  [unwired: 9 in, 1 out]
            }
            n180 = property on="数据写入成功" class="Bool (严格)"("Val(Sgnl)"=FALSE) -> ()  [unwired: 2 in, 2 out]
            n181 = property on="print_calibration" class="Bool (严格)"("DisabledEnum"=T1."Disabled and Grayed Out" ("禁用")) -> ()  [unwired: 2 in, 2 out]
            n182 = call-dynamic "Print Report.vi"("report in"=w487, "error in (no error)"=w488) -> ("report out"=w485:refnum<class "NI_report.lvclass">, "error out"=w486:errorcluster)  [unwired: 12 in]
            n183 = call-dynamic "Dispose Report.vi"("report in"=w485, "error in (no error)"=w486) -> ("error out"=w482:errorcluster)  [unwired: 13 in]
          }
        }
      }
      event "停止": Mouse Up {
        w511 = FALSE
        w513 = T1."Disabled and Grayed Out" ("禁用")
        n184 = event-data() -> ()  [unwired: 1 in, 1 out]
        n185 = property on="init" class="Bool (严格)"("Visible"=TRUE) -> ()  [unwired: 2 in, 2 out]
        n186 = property on="print_calibration" class="Bool (严格)"("DisabledEnum"=w513, "Visible"=w511) -> ()  [unwired: 2 in, 2 out]
        n187 = property on="print_data" class="Bool (严格)"("DisabledEnum"=w513, "Visible"=w511) -> ()  [unwired: 2 in, 2 out]
        n188 = property on="执行状态" class="Bool (严格)"("Val(Sgnl)"=w511) -> ()  [unwired: 2 in, 2 out]
        n189 = local write "初始化成功"(w511) -> ()
        n190 = property on="write" class="Bool (严格)"("Visible"=w511) -> ()  [unwired: 2 in, 2 out]
        n191 = property on="数据写入成功" class="Bool (严格)"("Val(Sgnl)"=w511) -> ()  [unwired: 2 in, 2 out]
      }
    }
    "error out" <- w18
    "执行状态" <- TRUE
  }
  n192 = property on="print_calibration" class="Bool (严格)"("DisabledEnum"=w13, "Visible"=w10) -> ()  [unwired: 2 in, 2 out]
  n193 = property on="init" class="Bool (严格)"("Visible"=TRUE) -> ()  [unwired: 2 in, 2 out]
  n194 = property on="print_data" class="Bool (严格)"("DisabledEnum"=w13, "Visible"=w10) -> ()  [unwired: 2 in, 2 out]
